vi "Robot Global Data.vi"() -> ()   [LabVIEW 2020]
doc: "This global VI can contain as many global variables as you need. Place a control on the panel, give it a good name. To read or write to it from a VI, drag the icon to the diagram of that VI. You can also drag from the project. Click on the node to change which global you access. You shouldn't have multiple locations writing to a global or it will cause a race-condition."
uses:
  <vilib>/Rock Robotics/WPI/Camera/WPI_CameraImageSize.ctl
  <vilib>/Rock Robotics/WPI/DriverStation/WPI_DriverStationRobotMode2.ctl
  <vilib>/Rock Robotics/WPI/DriverStation/WPI_DriverStationAllianceInfo.ctl
panel:
  out "Rumble":sgl
  out "Pvolts":dbl
  out "Pressure":dbl
  out "Adjustment 2":dbl
  out "TxAdj":dbl
  out "ShooterSet2":dbl
  out "ShooterVel2":dbl
  out "IntakeOn?":bool
  out "Adjustment":dbl
  out "Alliance":T1
  out "MatchTime":dbl
  out "ShooterSet":dbl
  out "RightEncAvg":dbl
  out "LeftEncAvg":dbl
  out "POV2":i16=-1
  out "POV1":i16=-1
  out "AutoState":string
  out "Gyro Angle":dbl
  out "DriveENCreset":bool
  out "GyroReset":bool
  out "Right2Enc":dbl
  out "Right1Enc":dbl
  out "Left2Enc":dbl
  out "Left1Enc":dbl
  out "TDistance":dbl
  out "TurretPos":dbl
  out "ShooterVel":dbl
  out "RStick2":bool
  out "LStick2":bool
  out "Option2":bool
  out "Share2":bool
  out "RightBumper2":bool
  out "LeftBumper2":bool
  out "X2":bool
  out "Circle2":bool
  out "Triangle2":bool
  out "Square2":bool
  out "RightTrigger2":dbl
  out "LeftTrigger2":dbl
  out "RightY2":dbl
  out "RightX2":dbl
  out "LeftY2":dbl
  out "LeftX2":dbl
  out "RStick1":bool
  out "LStick1":bool
  out "Option1":bool
  out "Share1":bool
  out "Ty":dbl
  out "Tx":dbl
  out "Tv":dbl
  out "RightBumper1":bool
  out "LeftBumper1":bool
  out "X1":bool
  out "Circle1":bool
  out "Triangle1":bool
  out "Square1":bool
  out "RightTrigger1":dbl
  out "LeftTrigger1":dbl
  out "RightY1":dbl
  out "RightX1":dbl
  out "LeftY1":dbl
  out "LeftX1":dbl
  in  "Robot Mode":T2
  in  "image size":T3=enum."320x240"
  in  "Enable Vision":bool
  # "Joystick Inputs"
  # "Sensor Inputs"
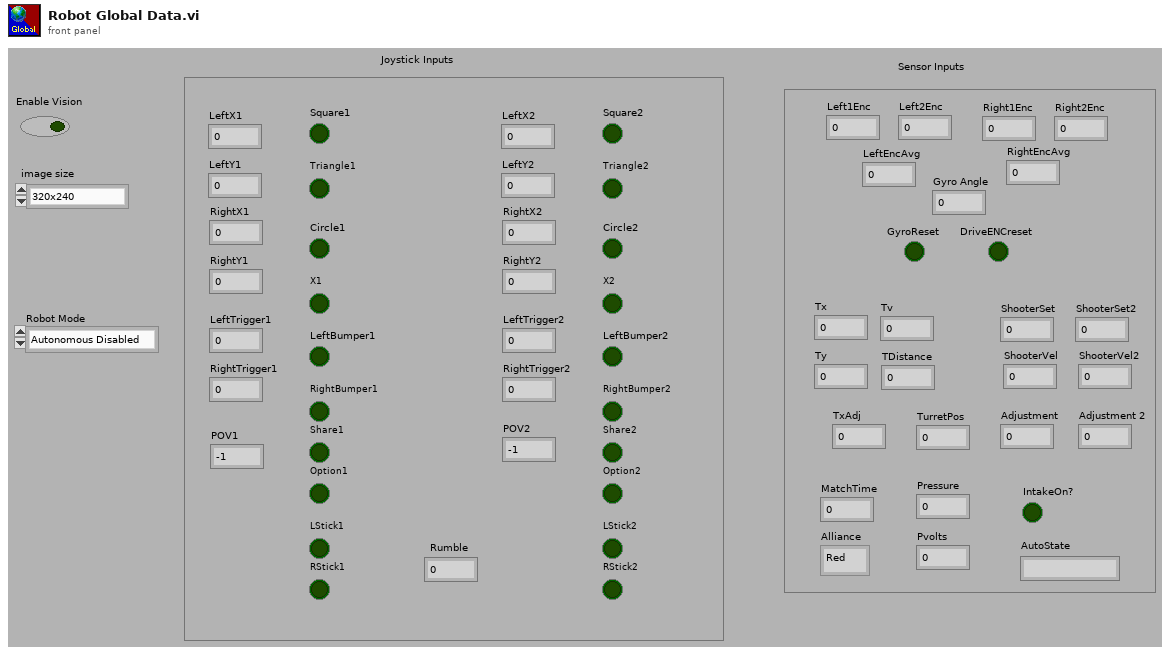
[diagram p1: front panel]
types:
  T1 = typedef "WPI_DriverStationAllianceInfo.ctl" = enum16{"Red", "Blue", "Invalid"}
  T2 = typedef "WPI_DriverStationRobotMode2.ctl" = enum16{"Autonomous Disabled", "Autonomous Enabled", "Teleop Disabled", "Teleop Enabled", "Disconnected", "Finish", "Test Disabled", "Test Enabled", "Emergency Stopped"}
  T3 = typedef "WPI_CameraImageSize.ctl" = enum16{"640x480", "320x240", "160x120", "Custom"}
diagram:
